vi "DIO mode set.vi"(8 "error in (no error)":errorcluster, 10 "mode":enum16{"input", "output"}(ring), 11 "DIO in":refnum<class "DIO.lvclass">) -> (0 "error out":errorcluster, 3 "DIO out":refnum<class "DIO.lvclass">)   [LabVIEW 2019, in "my FPGA lib.lvlib" / "DIO.lvclass"]
uses:
  DIO.lvclass
  DIO.lvclass/DIO.ctl
  <vilib>/Utility/error.llb/Error Cluster From Error Code.vi
  <vilib>/rvi/errors/niLvFpgaAdjustHostInterfaceError.vi
  <vilib>/rvi/interface/nirviReadWriteControl/nirviReadWriteControl.xnode
  NiFpgaLv.dll
  <vilib>/rvi/interface/Simulation/niFpgaSimulationCallBeginRW.vi
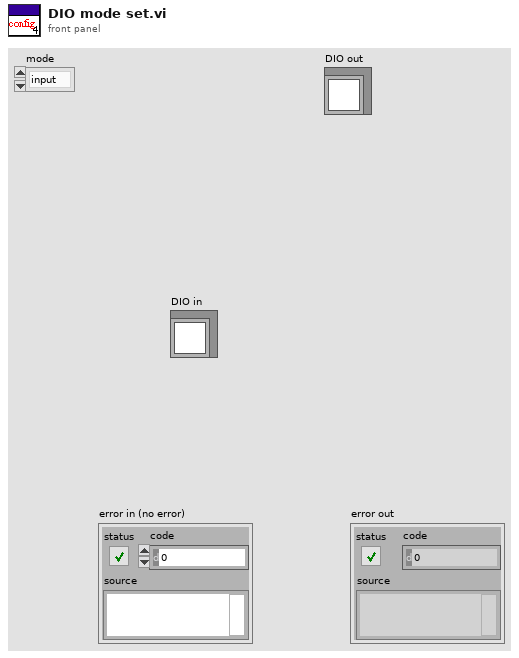
[diagram p1: front panel]
types:
  T1 = typedef "my FPGA lib.lvlib/DIO.lvclass/DIO enum.ctl" = enum16{"US.1", "US.2", "US.3", "US.4", "H.1", "H.2", "H.3", "H.4", "H.5"}
  T2 = typedef "my FPGA lib.lvlib/DIO.lvclass/port.ctl" = enum16{"US", "H."}
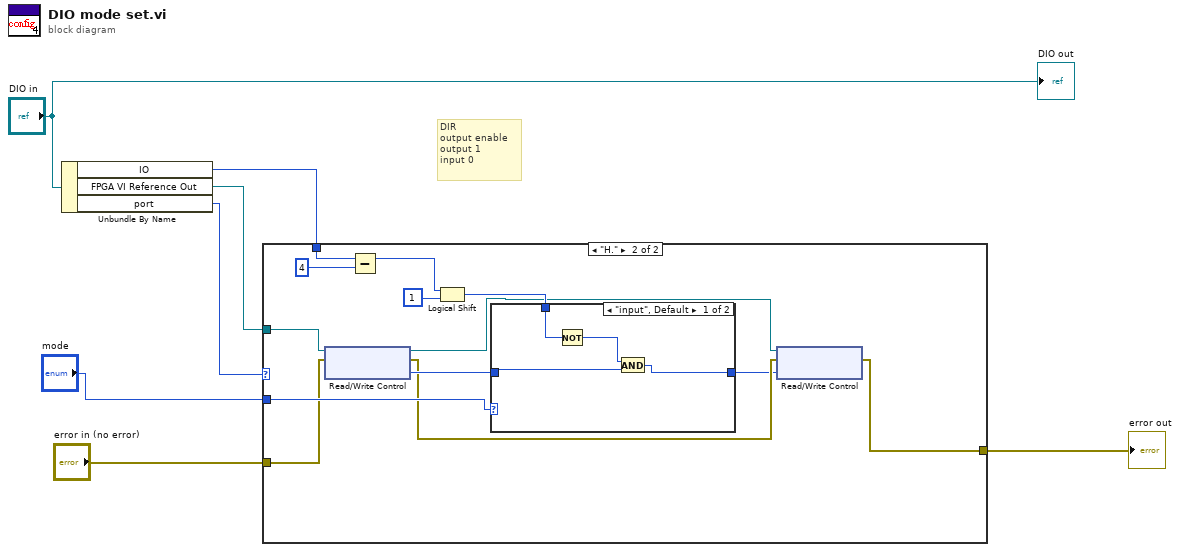
[diagram p0: block diagram]
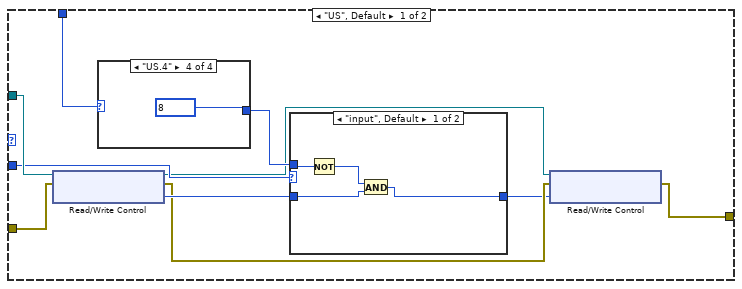
[diagram p2: hidden frame]
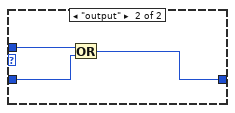
[diagram p3: hidden frame]
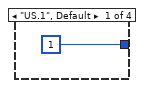
[diagram p4: hidden frame]
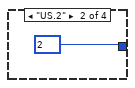
[diagram p5: hidden frame]
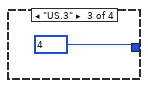
[diagram p6: hidden frame]
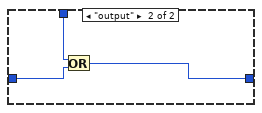
[diagram p7: hidden frame]
diagram:
  # "DIR\noutput enable\noutput 1\ninput 0"
  n1 = Unbundle By Name("DIO in") -> ("IO"=w5:T1, "FPGA VI Reference Out"=w3:refnum<k20>, "port"=w6:T2)
  n2 = case shown="\"H.\"" w6 {
    tunnel: w5 -> [w17 w40]
    tunnel: "error in (no error)" -> [w15 w37]
    tunnel: w3 -> [w16 w38]
    tunnel: "mode" -> [w14 w39]
    tunnel: [w8 w31] -> w1
    frame "US", Default {
      n3 = xnode "Read/Write Control"("FPGA VI Reference In"=w16, "error in"=w15) -> ("FPGA VI Reference Out"=w11:refnum<k20>, "error out"=w10:errorcluster, "Ultrasonic.io.DIR"=w12:u8)
      n4 = case shown="\"US.4\"" w17 {
        tunnel: [u8 1 u8 2 u8 4 u8 8] -> w13
        frame "US.1", Default {
        }
        frame "US.2" {
        }
        frame "US.3" {
        }
        frame "US.4" {
        }
      }
      n5 = case shown="\"input\", Default" w14 {
        tunnel: w13 -> [w21 w24]
        tunnel: w12 -> [w19 w23]
        tunnel: [w18 w22] -> w9
        frame "input", Default {
          n6 = Not(x=w21) -> (.not. x?=w20:u8)
          n7 = And(x=w20, y=w19) -> (x .and. y?=w18:u8)
        }
        frame "output" {
          n8 = Or(x=w24, y=w23) -> (x .or. y?=w22:u8)
        }
      }
      n9 = xnode "Read/Write Control"("FPGA VI Reference In"=w11, "error in"=w10, "Ultrasonic.io.DIR"=w9) -> ("error out"=w8:errorcluster)  [unwired: 1 out]
    }
    frame "H." {
      n10 = xnode "Read/Write Control"("FPGA VI Reference In"=w38, "error in"=w37) -> ("FPGA VI Reference Out"=w34:refnum<k20>, "error out"=w33:errorcluster, "Basic IO DIR"=w35:u8)
      n11 = Subtract(x=w40, y=4) -> (x-y=w30:i32)
      n12 = Logical Shift(y=w30, x=u8 1) -> (x << y=w36:u8)
      n13 = case shown="\"input\", Default" w39 {
        tunnel: w36 -> [w45 w48]
        tunnel: w35 -> [w43 w47]
        tunnel: [w42 w46] -> w32
        frame "input", Default {
          n14 = Not(x=w45) -> (.not. x?=w44:u8)
          n15 = And(x=w44, y=w43) -> (x .and. y?=w42:u8)
        }
        frame "output" {
          n16 = Or(x=w48, y=w47) -> (x .or. y?=w46:u8)
        }
      }
      n17 = xnode "Read/Write Control"("FPGA VI Reference In"=w34, "error in"=w33, "Basic IO DIR"=w32) -> ("error out"=w31:errorcluster)  [unwired: 1 out]
    }
  }
  "error out" <- w1
  "DIO out" <- "DIO in"
